vi "Rename_signals.vi"(8 "error in":errorcluster, 10 "Dynamic Data In":dynamicdata(waveform), 11 "New Signal Names":string[](array[string])=["SIGNAL_1", "SIGNAL_2", "SIGNAL3"]) -> (0 "error out":errorcluster, 3 "Dynamic Data Out":dynamicdata(waveform))   [LabVIEW 2025]
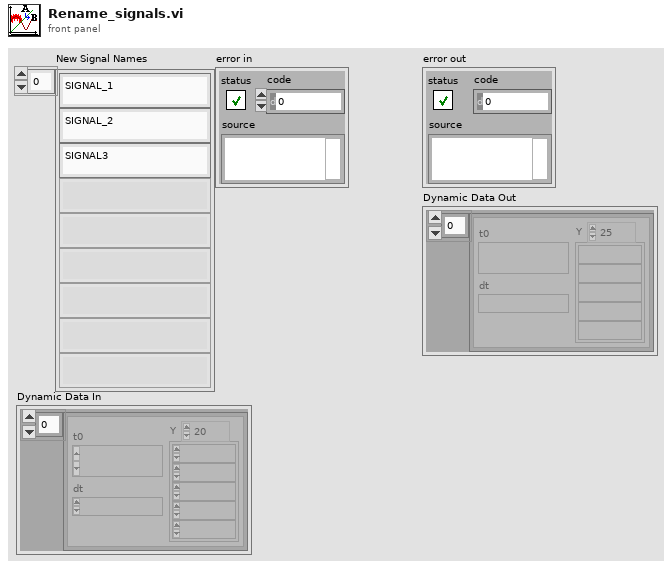
[diagram p1: front panel]
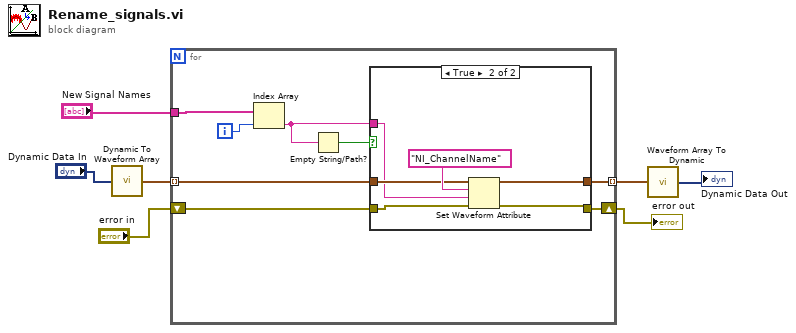
[diagram p0: block diagram]
diagram:
  n1 = call <vilib>:"Dynamic To Waveform Array.vi"("Input"="Dynamic Data In") -> ("Output"=w5:waveform(dbl)[])  [unwired: 4 in]
  n2 = for {
    tunnel: "New Signal Names" -> [w15]
    tunnel: w5 -> [w12] mode=indexing
    shift-right: [w10] -> w2
    shift-left: "error in" -> [w11]
    tunnel: [w9] -> w3 mode=indexing
    i -> [w14]
    n3 = Index Array(array=w15, index=w14) -> (element=w8:string)
    n4 = Empty String/Path?(string/path=w8) -> (empty?=w13:bool)
    n5 = case shown="True" w13 {
      tunnel: w12 -> [w17 w22]
      tunnel: w11 -> [w16 w21]
      tunnel: [w17 w20] -> w9
      tunnel: [w16 w19] -> w10
      tunnel: w8 -> [_ w18]
      frame False {
      }
      frame True {
        n6 = Set Waveform Attribute(4:w21, 5:w18, 6:"NI_ChannelName", 7:w22) -> (0:w19:errorcluster, 3:w20:waveform(dbl))  [unwired: 1 out]
      }
    }
  }
  "error out" <- w2
  n7 = call <vilib>:"Waveform Array To Dynamic.vi"("Input"=w3) -> ("Output"=→"Dynamic Data Out":dynamicdata)  [unwired: 4 in]
